vi "TCP - Client.vi"() -> ()   [LabVIEW 2019]
doc: "This VI implements a client for the TCP Named Service - Server.vi. It connects to a service by specifying the server address and the name of the service. The client receives the string sent by the server, displays the string and closes the connection."
panel:
  out "Waiting for Message":bool
  in  "Message to Server":string
  in  "SEND":bool
  out "Message from Server":string
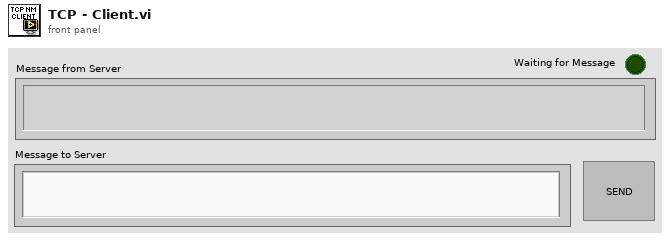
[diagram p1: front panel]
types:
  T1 = enum16{"Standard", "Buffered", "CRLF", "Immediate"}
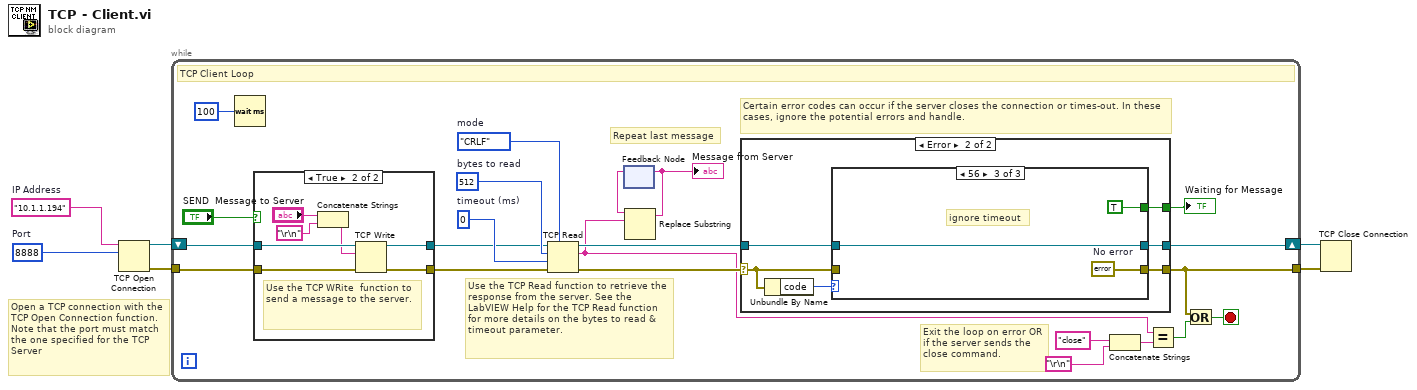
[diagram p0: block diagram]
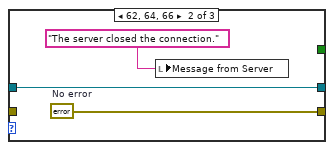
[diagram p5: hidden frame]
diagram:
  w4 = u16 8888  # Port
  w5 = "10.1.1.194"  # IP Address
  # "Open a TCP connection with the TCP Open Connection function. Note that the port must match the one specified for the TCP Server"
  n1 = TCP Open Connection(address=w5, remote port or service name=w4) -> (connection ID=w3:refnum<k5>, error out=w6:errorcluster)  [unwired: 3 in]
  n2 = while {
    tunnel: w6 -> [w16]
    shift-right: [w22] -> w1
    shift-left: w3 -> [w27]
    tunnel: [w13] -> w2
    stop <- w12 stop-if-true
    w18 = 0  # timeout (ms)
    w25 = T1."CRLF"  # mode
    w26 = 512  # bytes to read
    # "Repeat last message"
    # "Exit the loop on error OR if the server sends the close command."
    # "Use the TCP Read function to retrieve the response from the server. See the LabVIEW Help for the TCP Read function for more details on the bytes to read & timeout parameter."
    # "Certain error codes can occur if the server closes the connection or times-out. In these cases, ignore the potential errors and handle."
    # "TCP Client Loop"
    n3 = Wait (ms)(milliseconds to wait=u32 100) -> ()  [unwired: 1 out]
    n4 = case shown="True" "SEND" {
      tunnel: w27 -> [w30 w37]
      tunnel: [w30 w36] -> w17
      tunnel: w16 -> [w29 w35]
      tunnel: [w29 w34] -> w15
      frame False {
        # "Do nothing."
      }
      frame True {
        # "Use the TCP WRite  function to send a message to the server."
        n5 = Concatenate Strings("Message to Server", "\r\n") -> (w32:string)
        n6 = TCP Write(connection ID=w37, data in=w32, error in (no error)=w35) -> (connection ID out=w36:refnum<k5>, error out=w34:errorcluster)  [unwired: 1 in, 1 out]
      }
    }
    n7 = TCP Read(connection ID=w17, bytes to read=w26, error in (no error)=w15, 7:w25, 9:w18) -> (connection ID out=w23:refnum<k5>, data out=w10:string, error out=w24:errorcluster)
    n8 = feedback #1() -> (w8:string)  [unwired: 1 in]
    n9 = Replace Substring(4:w10, 5:w8) -> (1:w9:string)  [unwired: 2 in, 1 out]
    "Message from Server" <- w9
    n10 = feedback-in #1(w9) -> ()
    n11 = case shown="Error" w24 {
      selector: w24 -> [w39 w44]
      tunnel: [w39 w43] -> w13
      tunnel: w23 -> [w38 w42]
      tunnel: [w38 w41] -> w22
      tunnel: [_ w40] -> w7
      frame No Error {
      }
      frame Error {
        n12 = Unbundle By Name(w44) -> ("code"=w45:i32)
        n13 = case shown="56" w45 {
          tunnel: w44 -> [w47 _ _]
          tunnel: [w47 w50 w53] -> w43
          tunnel: [w46 w48 w52] -> w41
          tunnel: w42 -> [w46 w48 w52]
          tunnel: [_ _ TRUE] -> w40
          frame Default {
          }
          frame 62, 64, 66 {
            w50 = errorcluster {"status"=FALSE, "code"=0, "source"=""}  # No error
            n14 = local write "Message from Server"("The server closed the connection." ("Server Closed")) -> ()
          }
          frame 56 {
            w53 = errorcluster {"status"=FALSE, "code"=0, "source"=""}  # No error
            # "ignore timeout"
          }
        }
      }
    }
    "Waiting for Message" <- w7
    n15 = Concatenate Strings("close", "\r\n") -> (w20:string)
    n16 = Equal?(x=w10, y=w20) -> (x = y?=w11:bool)
    n17 = Or(x=w13, y=w11) -> (x .or. y?=w12:bool)
  }
  n18 = TCP Close Connection(connection ID=w1, error in (no error)=w2) -> ()  [unwired: 3 out]
